vi "GetBkData.vi"(0 "VISA resource name":refnum<visa-resource-name>, 5 "Mode":string, 7 "Value":string, 9 "Delay":string, 11 "error":errorcluster) -> (3 "Resistance":dbl, 4 "VISA resource name out":refnum<visa-resource-name>, 6 "Voltage":dbl, 8 "Current":dbl, 10 "Power":dbl, 14 "Setting":dbl, 15 "error out":errorcluster)   [LabVIEW 2010]
uses:
  <instrlib>/BK Precision 85XX Series/BK Precision 85XX Series.lvlib
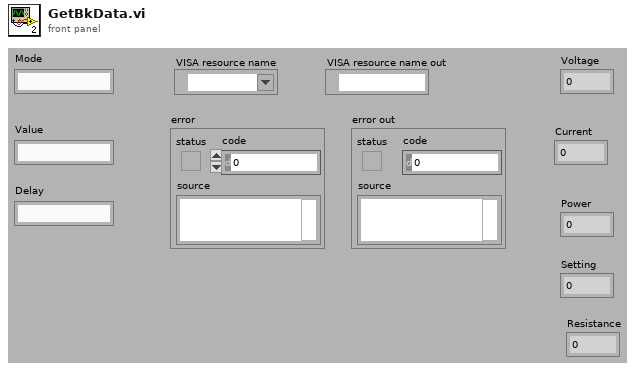
[diagram p1: front panel]
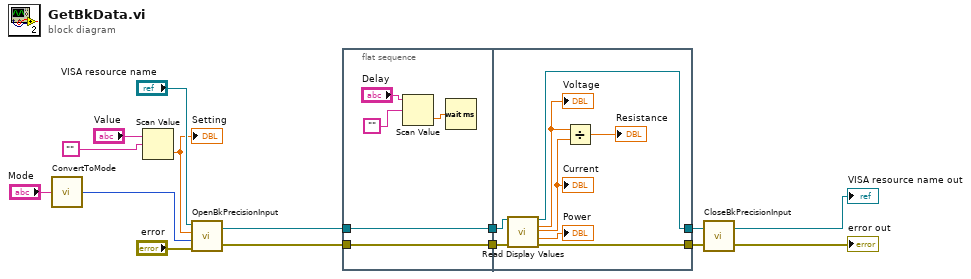
[diagram p0: block diagram]
diagram:
  n1 = call "ConvertToMode.vi"("String"="Mode") -> ("Numeric"=w9:i32)
  n2 = Scan Value(string="Value", format string="") -> (value=w2:dbl)  [unwired: 1 in, 1 out]
  "Setting" <- w2
  n3 = call "OpenBkPrecisionInput.vi"("error"="error", "Configuration State"=w9, "Configuration Value"=w2, "VISA resource name"="VISA resource name") -> ("error out 2"=w12:errorcluster, "VISA resource name"=w13:refnum<visa-resource-name>)
  n4 = flat-sequence {
    tunnel: w12 -> [w19]
    tunnel: w13 -> [w20]
    tunnel: [w20] -> w15
    tunnel: [w19] -> w14
    tunnel: w15 -> [w28]
    tunnel: w14 -> [w27]
    tunnel: [w26] -> w11
    tunnel: [w25] -> w10
    frame #0 {
      n5 = Scan Value(string="Delay", format string="") -> (value=w17:dbl)  [unwired: 1 in, 1 out]
      n6 = Wait (ms)(milliseconds to wait=w17) -> ()  [unwired: 1 out]
    }
    frame #1 {
      n7 = call <instrlib>:"Read Display Values.vi"("VISA resource name"=w28, "error in (no error)"=w27) -> ("VISA resource name out"=w26:refnum<visa-resource-name>, "Terminal Input Voltage (V)"=w22:dbl, "Terminal Input Current (A)"=w21:dbl, "Terminal Input Power (W)"=→"Power":dbl, "error out"=w25:errorcluster)  [unwired: 9 in]
      "Voltage" <- w22
      "Current" <- w21
      n8 = Divide(x=w22, y=w21) -> (x/y=→"Resistance":dbl)
    }
  }
  n9 = call "CloseBkPrecisionInput.vi"("error out 2"=w10, "VISA resource name out 2"=w11) -> ("error out"=→"error out":errorcluster, "VISA resource name out"=→"VISA resource name out":refnum<visa-resource-name>)
